vi "Parameter speed control.vi"(0 "Torque_Reference_LR":dbl, 1 "Engine Speed/moment LR":bool, 2 "L":sgl[](array[numeric]), 3 "R":sgl[](array[numeric]), 4 "Direction":bool, 5 "Output Ramp LR in":dbl, 6 "Ramp LR active":bool, 7 "Speed_Reference_LR":dbl, 11 "Numeric in":dbl, 12 "Mod6/Unit H":bool) -> (14 "Numeric 3":dbl, 15 "Output Ramp L out":dbl, 18 "Numeric out R":dbl)   [LabVIEW 2018]
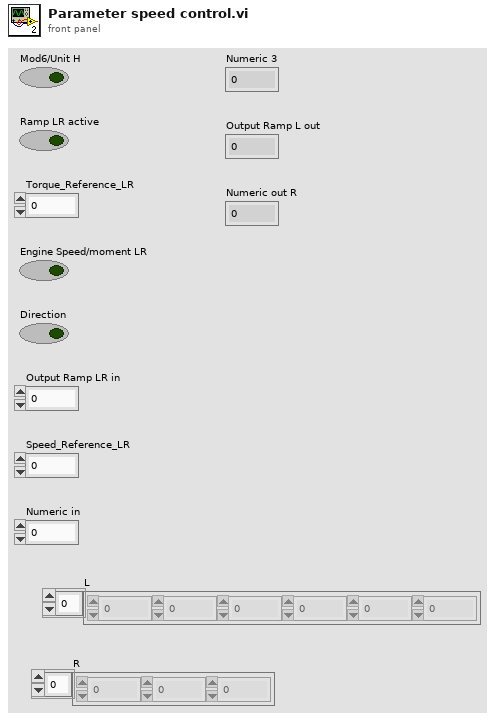
[diagram p1: front panel]
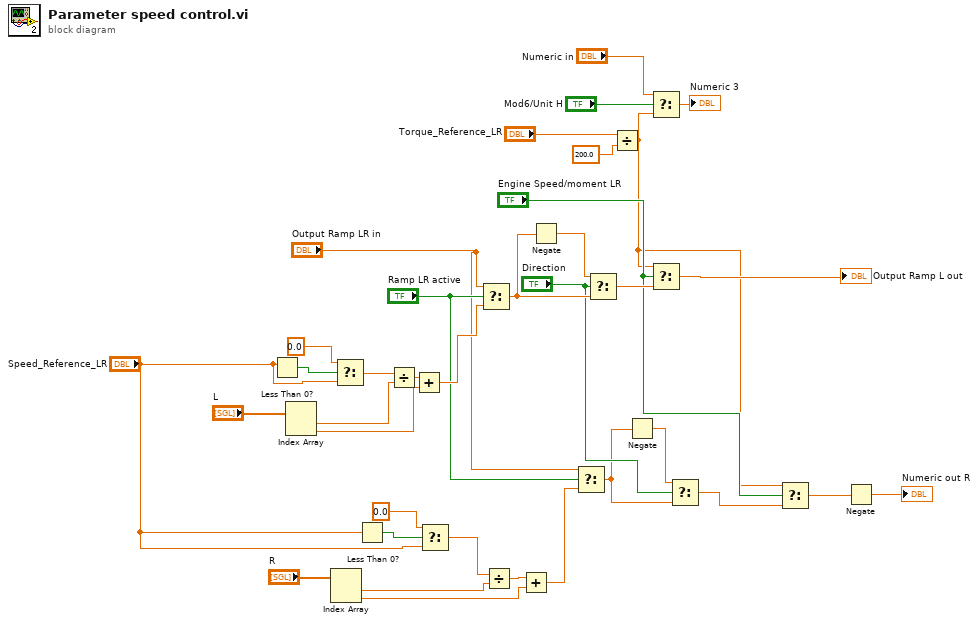
[diagram p0: block diagram]
diagram:
  n1 = Less Than 0?(x="Speed_Reference_LR") -> (x < 0?=w16:bool)
  n2 = Index Array(array="L") -> (element #1=w21:sgl, element #2=w20:sgl)  [unwired: 2 in]
  n3 = Index Array(array="R") -> (element #1=w24:sgl, element #2=w23:sgl)  [unwired: 2 in]
  n4 = Select(t=0.0, s=w16, f="Speed_Reference_LR") -> (s? t:f=w15:dbl)
  n5 = Less Than 0?(x="Speed_Reference_LR") -> (x < 0?=w12:bool)
  n6 = Divide(x=w15, y=w21) -> (x/y=w14:dbl)
  n7 = Add(x=w14, y=w20) -> (x+y=w29:dbl)
  n8 = Select(t=0.0, s=w12, f="Speed_Reference_LR") -> (s? t:f=w9:dbl)
  n9 = Select(t="Output Ramp LR in", s="Ramp LR active", f=w29) -> (s? t:f=w31:dbl)
  n10 = Divide(x=w9, y=w24) -> (x/y=w26:dbl)
  n11 = Add(x=w26, y=w23) -> (x+y=w8:dbl)
  n12 = Negate(x=w31) -> (-x=w27:dbl)
  n13 = Select(t="Output Ramp LR in", s="Ramp LR active", f=w8) -> (s? t:f=w5:dbl)
  n14 = Select(t=w27, s="Direction", f=w31) -> (s? t:f=w32:dbl)
  n15 = Divide(x="Torque_Reference_LR", y=200.0) -> (x/y=w3:dbl)
  n16 = Negate(x=w5) -> (-x=w6:dbl)
  n17 = Select(t="Numeric in", s="Mod6/Unit H", f=w3) -> (s? t:f=→"Numeric 3":dbl)
  n18 = Select(t=w3, s="Engine Speed/moment LR", f=w32) -> (s? t:f=→"Output Ramp L out":dbl)
  n19 = Select(t=w6, s="Direction", f=w5) -> (s? t:f=w2:dbl)
  n20 = Select(t=w3, s="Engine Speed/moment LR", f=w2) -> (s? t:f=w1:dbl)
  n21 = Negate(x=w1) -> (-x=→"Numeric out R":dbl)
